vi "GEOM_ReadFPA.vi"(6 "override format":string, 7 "moddir":path=path "/kkk", 8 "error in (no error)":errorcluster, 9 "Database RefNum out":T1, 10 "FPA":string, 11 "database path":path=path "/home/ArcVIEW/Modules/GEOM/public/database") -> (0 "error out":errorcluster, 1 "FPAReadModes":T14[](array[typedef]) {"Amplifiers"."fliped" items=["none", "horizontal", "vertical"]; "Amplifiers"."type" items=["LL", "LR", "UL", "UR"]}, 2 "FPA":T10 {"Sorted Detectors"."ReadModes"."amplifiers"."fliped" items=["none", "horizontal", "vertical"]; "Sorted Detectors"."ReadModes"."amplifiers"."type" items=["LL", "LR", "UL", "UR"]}, 3 "database path out":path=path "/home/ArcVIEW/Modules/Geometry/database/TYPES/Hawaii-II_4ch.chp", 4 "modifiers":T11={"Binning"={"x"=1, "y"=1}, "sections"=[]} {"Binning"."y" min=1; "Binning"."x" min=1}, 5 "detreadmodes":cluster{"name":string, "detectors":T2[]}[](array[cluster]))   [LabVIEW 2016]
uses:
  GEOM_FPAReadMode.ctl
  GEOM_Amplifier.ctl
  GEOM_AmpType.ctl
  GEOM_ROI.ctl
  GEOM_Coords.ctl
  GEOM_AmpModifiers.ctl
  GEOM_Binning.ctl
  GEOM_Moifier.ctl
  GEOM_FPADetectors.ctl
  GEOM_DetStruct.ctl
  GEOM_ReadMode.ctl
  GEOM_DetSummaryStruct.ctl
  DBSHAND/private/vis/DatabaseHand_RefNum.ctl
  GEOM_VAR_action.ctl
  <vilib>/Utility/config.llb/Read Key (String).vi
  DBSHAND/private/vis/DatabaseHand_Element_Set(string).vi
  <vilib>/Utility/config.llb/NI_LVConfig.lvlib
panel:
  in  "Detector":T3 {"ReadModes"."amplifiers"."fliped" items=["none", "horizontal", "vertical"]; "ReadModes"."amplifiers"."type" items=["LL", "LR", "UL", "UR"]}
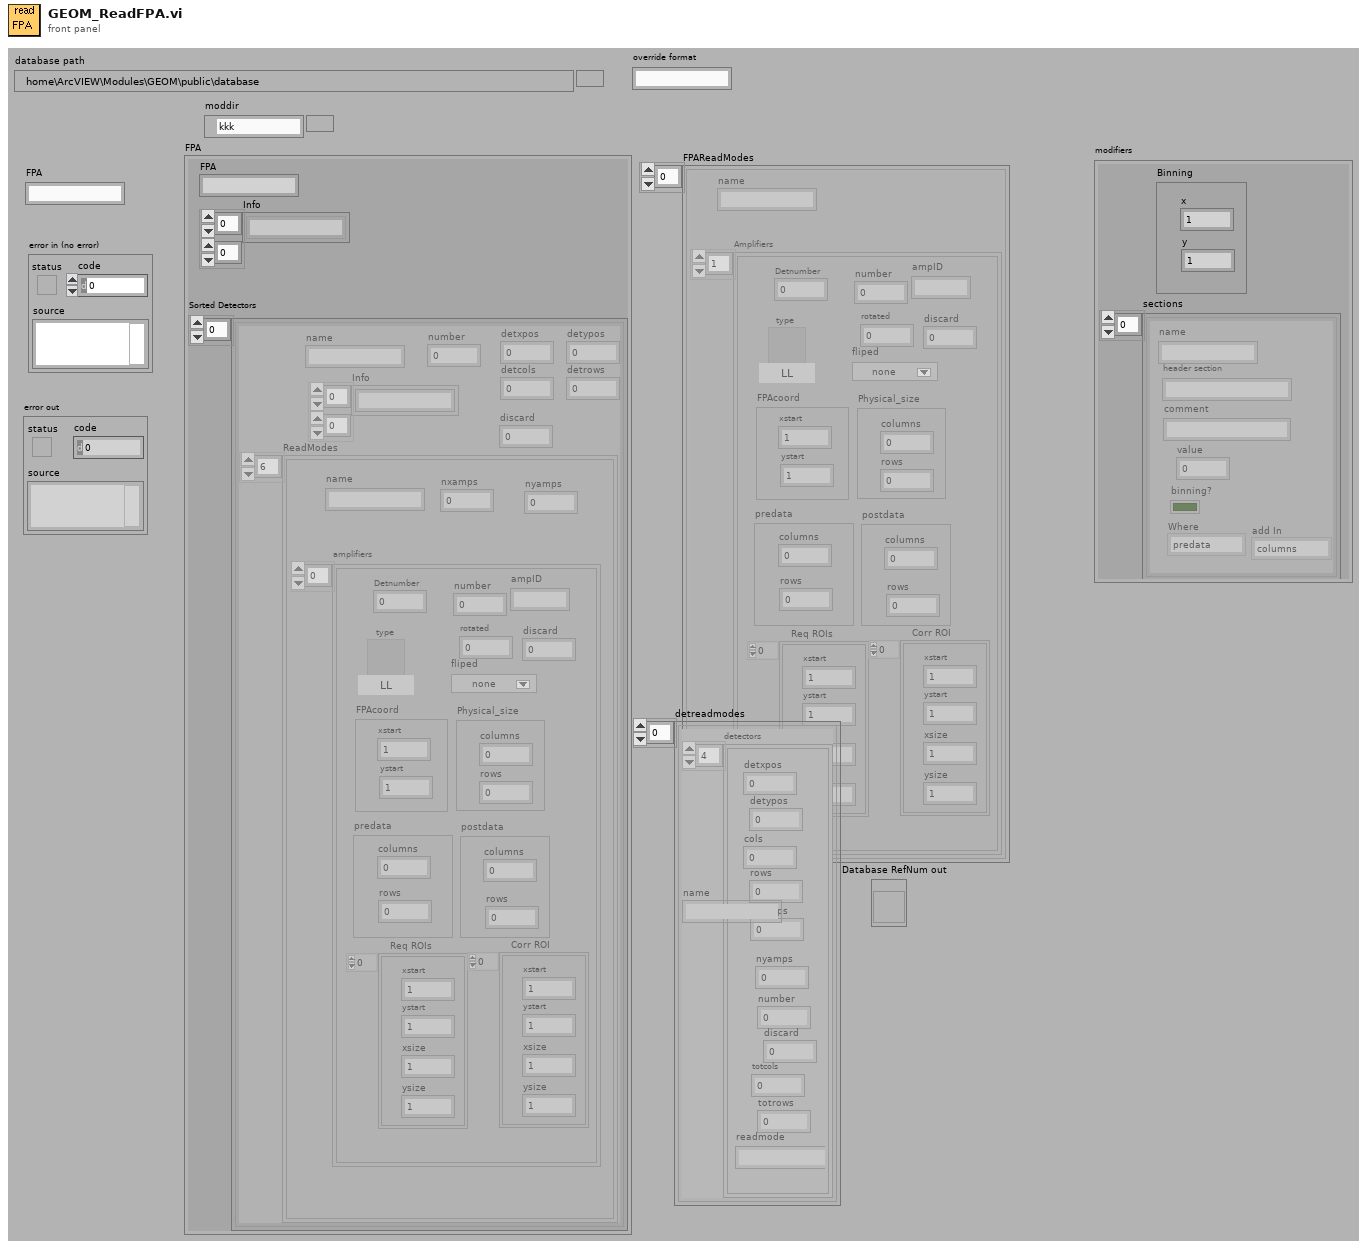
[diagram p1: front panel]
types:
  T1 = typedef "DatabaseHand_RefNum.ctl" = refnum<vi>
  T2 = typedef "GEOM_DetSummaryStruct.ctl" = cluster{"detxpos":i32, "detypos":i32, "cols":i32, "rows":i32, "nxamps":i32, "nyamps":i32, "number":i32, "discard":i32, "totcols":i32, "totrows":i32, "readmode":string}
  T3 = typedef "GEOM_DetStruct.ctl" = cluster{"name":string, "number":i32, "Info":string[][], "ReadModes":T4[], "detxpos":i32, "detypos":i32, "detcols":i32, "detrows":i32, "discard":i32}
  T4 = typedef "GEOM_ReadMode.ctl" = cluster{"name":string, "amplifiers":T5[], "nxamps":i32, "nyamps":i32}
  T5 = typedef "GEOM_Amplifier.ctl" = cluster{"number":i32, "type":T6, "rotated":i16, "fliped":u16, "FPAcoord":cluster{"xstart":i32, "ystart":i32}, "Physical_size":cluster{"columns":i32, "rows":i32}, "predata":cluster{"columns":i32, "rows":i32}, "postdata":cluster{"columns":i32, "rows":i32}, "Req ROIs":T7, "Corr ROI":T7, "Detnumber":i32, "ampID":string, "discard":i32}
  T6 = typedef "GEOM_AmpType.ctl" = u16
  T7 = typedef "GEOM_ROI.ctl" = T8[]
  T8 = typedef "GEOM_Coords.ctl" = cluster{"xstart":u32, "ystart":u32, "xsize":u32, "ysize":u32}
  T9 = typedef "GEOM_FPADetectors.ctl" = T3[]
  T10 = cluster{"FPA":string, "Info":string[][], "Sorted Detectors":T9}
  T11 = typedef "GEOM_AmpModifiers.ctl" = cluster{"Binning":T12, "sections":T13[]}
  T12 = typedef "GEOM_Binning.ctl" = cluster{"x":u32, "y":u32}
  T13 = typedef "GEOM_Moifier.ctl" = cluster{"name":string, "header section":string, "comment":string, "value":i32, "binning?":bool, "Where":enum16{"predata", "postdata"}, "add In":enum16{"columns", "rows", "none"}}
  T14 = typedef "GEOM_FPAReadMode.ctl" = cluster{"name":string, "Amplifiers":T5[]}
  T15 = typedef "NI_LVConfig.lvlib/Config Data RefNum.ctl" = refnum<k1>
  T16 = typedef "GEOM_VAR_action.ctl" = enum16{"read", "write"}
  T17 = cluster{"name":string, "Info":string[][], "ReadModes":T4[]}
  T18 = cluster{"name":string, "ReadType":string, string[]}[]
  T19 = cluster{"name":string, "Info":string[][], "Sorted Detectors":T9}
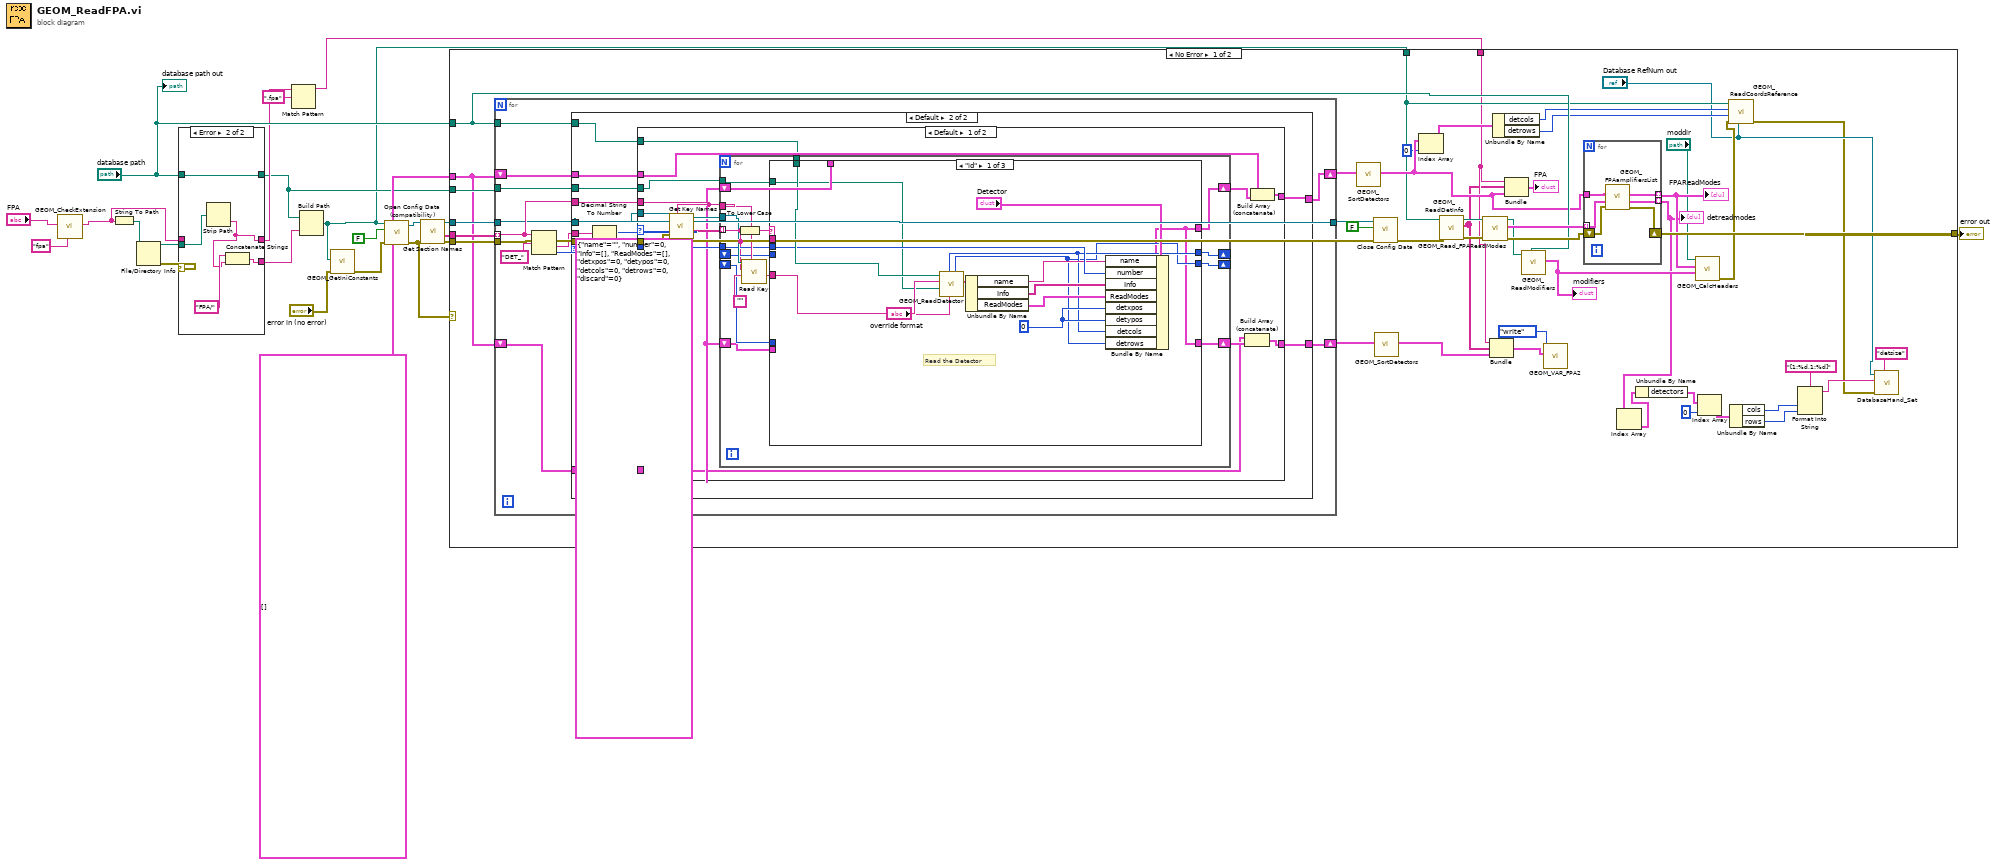
[diagram p0: block diagram]
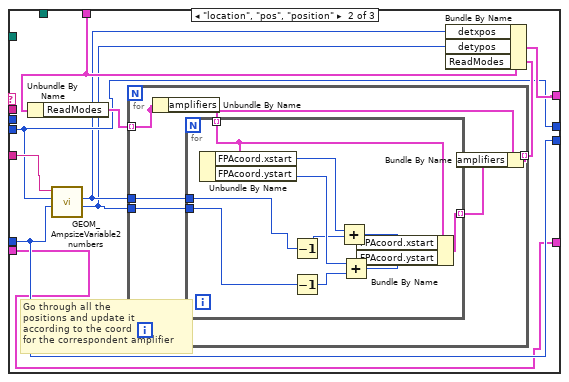
[diagram p3: hidden frame]
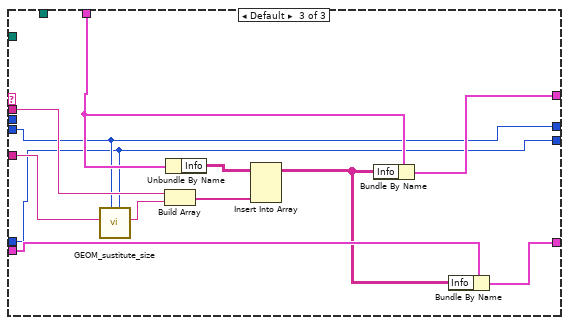
[diagram p4: hidden frame]
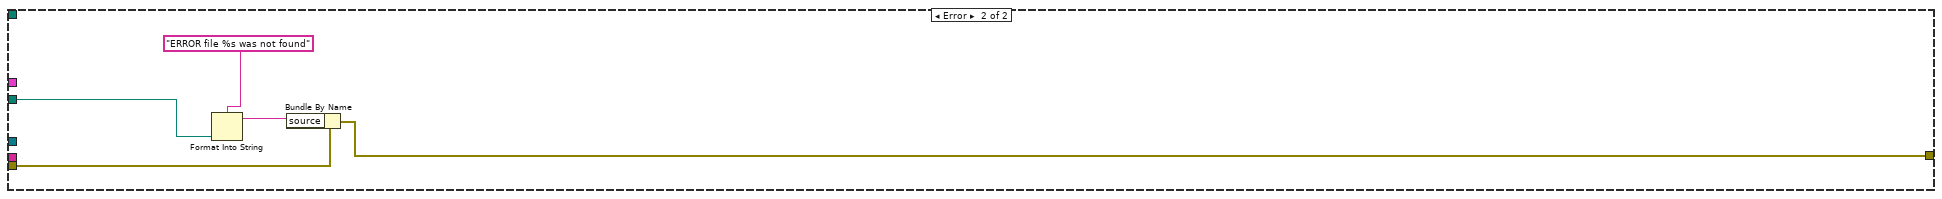
[diagram p6: hidden frame]
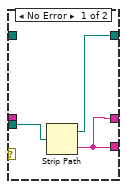
[diagram p7: hidden frame]
diagram:
  n1 = call "GEOM_CheckExtension.vi"("extension to look"="fpa", "name in"="FPA") -> ("name out"=w11:string)  [unwired: 8 out]
  n2 = String To Path(string=w11) -> (path=w17:path)
  n3 = File/Directory Info(path=w17) -> (path out=w14:path, error out=w16:errorcluster)  [unwired: 1 in, 5 out]
  n4 = case shown="Error" w16 {
    tunnel: w11 -> [_ _]
    tunnel: [w26 w27] -> w10
    tunnel: [w26 w30] -> w15
    tunnel: w14 -> [w25 w28]
    tunnel: "database path" -> [_ w29]
    tunnel: [w24 w29] -> w5
    frame No Error {
      n5 = Strip Path(path=w25) -> (stripped path=w24:path, name=w26:string)
    }
    frame Error {
      n6 = Strip Path(path=w28) -> (name=w27:string)  [unwired: 1 out]
      n7 = Concatenate Strings("FPA/" ("string"), w27) -> (w30:string)
    }
  }
  n8 = Match Pattern(string=w10, regular expression=".fpa") -> (before substring=w6:string)  [unwired: 4 out]
  n9 = Build Path(base path=w5, name or relative path=w15) -> (appended path=w3:path)
  n10 = call "GEOM_GetIniConstants.vi"("error in (no error)"="error in (no error)", "fpa  file"=w3) -> ("error out"=w1:errorcluster)  [unwired: 9 out]
  n11 = call <vilib>:"Open Config Data (compatibility).vi"("error in (no error)"=w1, "create file if necessary (T)"=FALSE ("create file if necessary? (T)"), "configuration file path"=w3) -> ("error out"=w7:errorcluster, "refnum"=w20:T15)  [unwired: 6 in, 1 out]
  n12 = call <vilib>:"Get Section Names.vi"("error in (no error)"=w7, "refnum"=w20) -> ("error out"=w18:errorcluster, "section names"=w21:string[], "refnum out"=w22:T15)  [unwired: 7 out]
  n13 = case shown="No Error" w7 {
    tunnel: w22 -> [w76 _]
    tunnel: w21 -> [w75 _]
    tunnel: [w70 w195] -> w19
    tunnel: w18 -> [w69 w199]
    tunnel: w5 -> [w61 w196]
    tunnel: w3 -> [w53 _]
    tunnel: "database path" -> [w59 _]
    tunnel: w6 -> [w50 _]
    tunnel: T3[] [] -> [w52 _]
    frame No Error {
      n14 = for {
        tunnel: w76 -> [w89]
        tunnel: w75 -> [w91] mode=indexing
        shift-right: [w87] -> w64
        shift-left: w52 -> [w90]
        tunnel: [w89] -> w68
        tunnel: w69 -> [w88]
        tunnel: w61 -> [w86]
        tunnel: w59 -> [w85]
        shift-right: [w84] -> w51
        shift-left: w52 -> [w83]
        n15 = Match Pattern(string=w91, regular expression="DET_") -> (after substring=w92:string, offset past match=w93:i32)  [unwired: 3 out]
        n16 = case shown="Default" w93 {
          tunnel: w92 -> [_ w108]
          tunnel: w91 -> [_ w106]
          tunnel: w89 -> [_ w105]
          tunnel: [w96 w103] -> w87
          tunnel: w90 -> [w96 w100]
          tunnel: w88 -> [_ w102]
          tunnel: w86 -> [_ w101]
          tunnel: w85 -> [_ w99]
          tunnel: [w95 w98] -> w84
          tunnel: w83 -> [w95 w97]
          frame -1 {
          }
          frame Default {
            n17 = Decimal String To Number(string=w108) -> (offset past number=w107:i32, number=w104:i32)  [unwired: 2 out]
            n18 = case shown="Default" w107 {
              tunnel: w106 -> [w121 _]
              tunnel: w105 -> [w123 _]
              tunnel: w104 -> [w117 _]
              tunnel: [w118 w194] -> w103
              tunnel: w102 -> [w119 _]
              tunnel: w101 -> [w116 _]
              tunnel: w100 -> [w114 w194]
              tunnel: w99 -> [w113 _]
              tunnel: [w111 w193] -> w98
              tunnel: w97 -> [w109 w193]
              frame Default {
                w110 = T3 {"name"="", "number"=0, "Info"=[], "ReadModes"=[], "detxpos"=0, "detypos"=0, "detcols"=0, "detrows"=0, "discard"=0} ("Detector")
                n19 = call <vilib>:"Get Key Names.vi"("section"=w121, "error in (no error)"=w119, "refnum"=w123) -> ("key names"=w122:string[], "refnum out"=w120:T15)  [unwired: 7 out]
                n20 = for {
                  tunnel: w122 -> [w124] mode=indexing
                  tunnel: w121 -> [w139]
                  tunnel: w120 -> [w136]
                  tunnel: w117 -> [w135]
                  tunnel: w116 -> [w134]
                  shift-right: [w133] -> w115
                  shift-left: w110 -> [w132]
                  shift-right: [w131] -> _
                  shift-left: _ -> [w129]
                  shift-right: [w130] -> _
                  shift-left: _ -> [w128]
                  tunnel: w113 -> [w127]
                  shift-right: [w126] -> w112
                  shift-left: w110 -> [w125]
                  n21 = To Lower Case(string=w124) -> (all lower case string=w140:string)
                  n22 = call-poly <vilib>:"Read Key.vi"("section"=w139, "default value"="", "key"=w124, "refnum"=w136) -> ("value"=w137:string)  [unwired: 2 in, 5 out]
                  n23 = case shown="\"id\"" w140 {
                    tunnel: w137 -> [w153 w160 w184]
                    tunnel: w135 -> [w149 _ _]
                    tunnel: w134 -> [w142 _ _]
                    tunnel: [w141 w161 w186] -> w133
                    tunnel: w132 -> [_ w162 w187]
                    tunnel: [w144 w159 w182] -> w131
                    tunnel: [w143 w158 w181] -> w130
                    tunnel: w129 -> [_ w159 w182]
                    tunnel: w128 -> [_ w158 w181]
                    tunnel: w127 -> [w151 _ _]
                    tunnel: [w141 w155 w191] -> w126
                    tunnel: w125 -> [_ w155 w192]
                    tunnel: w124 -> [_ _ w190]
                    frame "id" {
                      w145 = 0
                      # "Read the Detector"
                      n24 = call "GEOM_ReadDetector.vi"("override format"="override format", "detectors path"=w142, "Detector Name"=w153, "database path"=w151) -> ("Detector"=w154:T17, "ydata"=w143:i32, "xdata"=w144:i32)  [unwired: 1 in, 4 out]
                      n25 = Unbundle By Name(w154) -> ("name"=w146:string, "Info"=w147:string[][], "ReadModes"=w148:T4[])
                      n26 = Bundle By Name(cluster="Detector", "name"=w146, "number"=w149, "Info"=w147, "ReadModes"=w148, "detxpos"=w145, "detypos"=w145, "detcols"=w144, "detrows"=w143) -> (w141:T3)
                    }
                    frame "location", "pos", "position" {
                      # "Go through all the\npositions and update it\naccording to the coord\nfor the correspondent amplifier"
                      n27 = Unbundle By Name(w162) -> ("ReadModes"=w164:T4[])
                      n28 = call "GEOM_AmpsizeVariable2numbers.vi"("detrows"=w158, "detcols"=w159, "ampval"=w160) -> ("amprows"=w156:i32, "ampcols"=w157:i32)  [unwired: 1 in, 6 out]
                      n29 = for {
                        tunnel: w164 -> [w168] mode=indexing
                        tunnel: [w167] -> w163 mode=indexing
                        tunnel: w157 -> [w166]
                        tunnel: w156 -> [w165]
                        n30 = Unbundle By Name(w168) -> ("amplifiers"=w170:T5[])
                        n31 = for {
                          tunnel: [w176] -> w169 mode=indexing
                          tunnel: w170 -> [w175] mode=indexing
                          tunnel: w166 -> [w172]
                          tunnel: w165 -> [w171]
                          n32 = Unbundle By Name(w175) -> ("FPAcoord.xstart"=w180:i32, "FPAcoord.ystart"=w179:i32)
                          n33 = Decrement(x=w172) -> (x-1=w173:i32)
                          n34 = Decrement(x=w171) -> (x-1=w174:i32)
                          n35 = Add(x=w180, y=w173) -> (x+y=w178:i32)
                          n36 = Add(x=w179, y=w174) -> (x+y=w177:i32)
                          n37 = Bundle By Name(cluster=w175, "FPAcoord.xstart"=w178, "FPAcoord.ystart"=w177) -> (w176:T5)
                        }
                        n38 = Bundle By Name(cluster=w168, "amplifiers"=w169) -> (w167:T4)
                      }
                      n39 = Bundle By Name(cluster=w162, "detxpos"=w157, "detypos"=w156, "ReadModes"=w163) -> (w161:T3)
                    }
                    frame Default {
                      n40 = call "GEOM_sustitute_size.vi"("detrows"=w181, "detcols"=w182, "info str"=w184) -> ("info str out"=w183:string)  [unwired: 8 out]
                      n41 = Build Array(w190, w183) -> (w188:string[])
                      n42 = Unbundle By Name(w187) -> ("Info"=w189:string[][])
                      n43 = Insert Into Array(array=w189, new element=w188) -> (w185:string[][])  [unwired: 2 in]
                      n44 = Bundle By Name(cluster=w187, "Info"=w185) -> (w186:T3)
                      n45 = Bundle By Name(cluster=w192, "Info"=w185) -> (w191:T3)
                    }
                  }
                }
                n46 = Build Array (concatenate)(w109, w112) -> (w111:T3[])
                n47 = Build Array (concatenate)(w114, w115) -> (w118:T3[])
              }
              frame -1 {
              }
            }
          }
        }
      }
      n48 = call "GEOM_SortDetectors.vi"("Detectors"=w64) -> ("Sorted Detectors"=w58:T9)  [unwired: 10 out]
      n49 = call <vilib>:"Close Config Data.vi"("error in (no error)"=w69, "write file if changed (T)"=FALSE ("write configuration file? (T)"), "refnum"=w68) -> ("error out"=w55:errorcluster)  [unwired: 8 out]
      n50 = call "GEOM_SortDetectors.vi"("Detectors"=w51) -> ("Sorted Detectors"=w48:T9)  [unwired: 10 out]
      n51 = Index Array(array=w58, index=0) -> (element=w56:T3)
      n52 = call "GEOM_ReadDetInfo.vi"("error in (no error)"=w55, "file path"=w53) -> ("error out"=w74:errorcluster, "Info"=w49:string[][], "file path out"=w73:path)  [unwired: 7 out]
      n53 = call "GEOM_Read_FPAReadModes.vi"("error in (no error)"=w74, "file path"=w73) -> ("error out"=w71:errorcluster, "FPAReadModes"=w72:T18, "file path out"=w60:path)  [unwired: 7 out]
      n54 = Bundle("name"=w50, "Info"=w49, "Sorted Detectors"=w48) -> (w47:T19)  [unwired: 1 out]
      n55 = Unbundle By Name(w56) -> ("detcols"=w45:i32, "detrows"=w44:i32)
      n56 = Bundle("name"=w50, "Info"=w49, "Sorted Detectors"=w58) -> (→"FPA":T19)  [unwired: 1 out]
      n57 = call "GEOM_ReadModifiers.vi"("database path"=w59, "fpa file"=w60) -> ("modifiers"=w65:T11)  [unwired: 1 in, 8 out]
      "modifiers" <- w65
      n58 = call "GEOM_VAR_FPA2.vi"("Action"=GEOM_VAR_action."write", "GEOM_FPA"=w47) -> ()  [unwired: 10 out]
      n59 = for {
        tunnel: w58 -> [w82]
        tunnel: w72 -> [w78] mode=indexing
        shift-right: [w80] -> w70
        shift-left: w71 -> [w81]
        tunnel: [w79] -> w66 mode=indexing
        tunnel: [w77] -> w32 mode=indexing
        n60 = call "GEOM_FPAamplifiersList.vi"("error in (no error)"=w81, "FPAReadMode"=w78, "Detectors"=w82) -> ("error out"=w80:errorcluster, "detreadmode"=w77:cluster{"name":string, "detectors":T2[]}, "FPAReadMode 2"=w79:T14)  [unwired: 6 out]
      }
      "FPAReadModes" <- w66
      "detreadmodes" <- w32
      n61 = Index Array(array=w32) -> (element=w35:cluster{"name":string, "detectors":T2[]})  [unwired: 1 in]
      n62 = Unbundle By Name(w35) -> ("detectors"=w40:T2[])
      n63 = call "GEOM_CalcHeaders.vi"("modifiers"=w65, "FPAReadModes"=w66, "moddir"="moddir") -> ("error out"=w54:errorcluster)  [unwired: 1 in, 7 out]
      n64 = Index Array(array=w40, index=0) -> (element=w38:T2)
      n65 = call "GEOM_ReadCoordsReference.vi"("Database RefNum in"="Database RefNum out", "error in (no error)"=w54, "detrows"=w44, "detcols"=w45, "file path"=w53) -> ("error out"=w33:errorcluster)  [unwired: 6 out]
      n66 = Unbundle By Name(w38) -> ("cols"=w37:i32, "rows"=w36:i32)
      n67 = Format Into String(format string="[1:%d,1:%d]", w37, w36) -> (resulting string=w41:string)  [unwired: 2 in, 1 out]
      n68 = call-poly "DatabaseHand_Set.vi"("name"="detsize", "error in (no error)"=w33, "value"=w41, "Database RefNum in"="Database RefNum out") -> ()  [unwired: 4 in, 4 out]
    }
    frame Error {
      n69 = Format Into String(format string="ERROR file %s was not found" ("source"), w196) -> (resulting string=w197:string)  [unwired: 2 in, 1 out]
      n70 = Bundle By Name(cluster=w199, "source"=w197) -> (w195:errorcluster)
    }
  }
  "error out" <- w19
  "database path out" <- "database path"
